vi "Gaussian.vi"() -> ()   [LabVIEW 2011]
uses:
  <vilib>/Math Plots/2D Math Plots/2D Error Bar/2D Error Bar XCtrl/2D Error Bar.xctl
  <vilib>/Math Plots/2D Math Plots/2D Error Bar/2D Error Bar Datatype/Public/Plot Helper (Fixed).vi
  <vilib>/Math Plots/2D Math Plots/2D Error Bar/2D Error Bar Datatype/Public/Plot Helper (Percentage).vi
  <vilib>/Analysis/NI_AALPro.lvlib
  <vilib>/Math Plots/2D Math Plots/2D Error Bar/2D Error Bar Datatype/2D Error Bar Datatype.lvclass
panel:
  in  "y-error (or above)":dbl[](array[numeric])
  in  "x-error (or below)":dbl[](array[numeric])
  out "2D Error Bar":refnum<class "2D Plot Datatype.lvclass">[](xcontrol)
  in  "Array - Numeric":dbl[][](array[numeric])
  out "XY Graph":T1(graph)
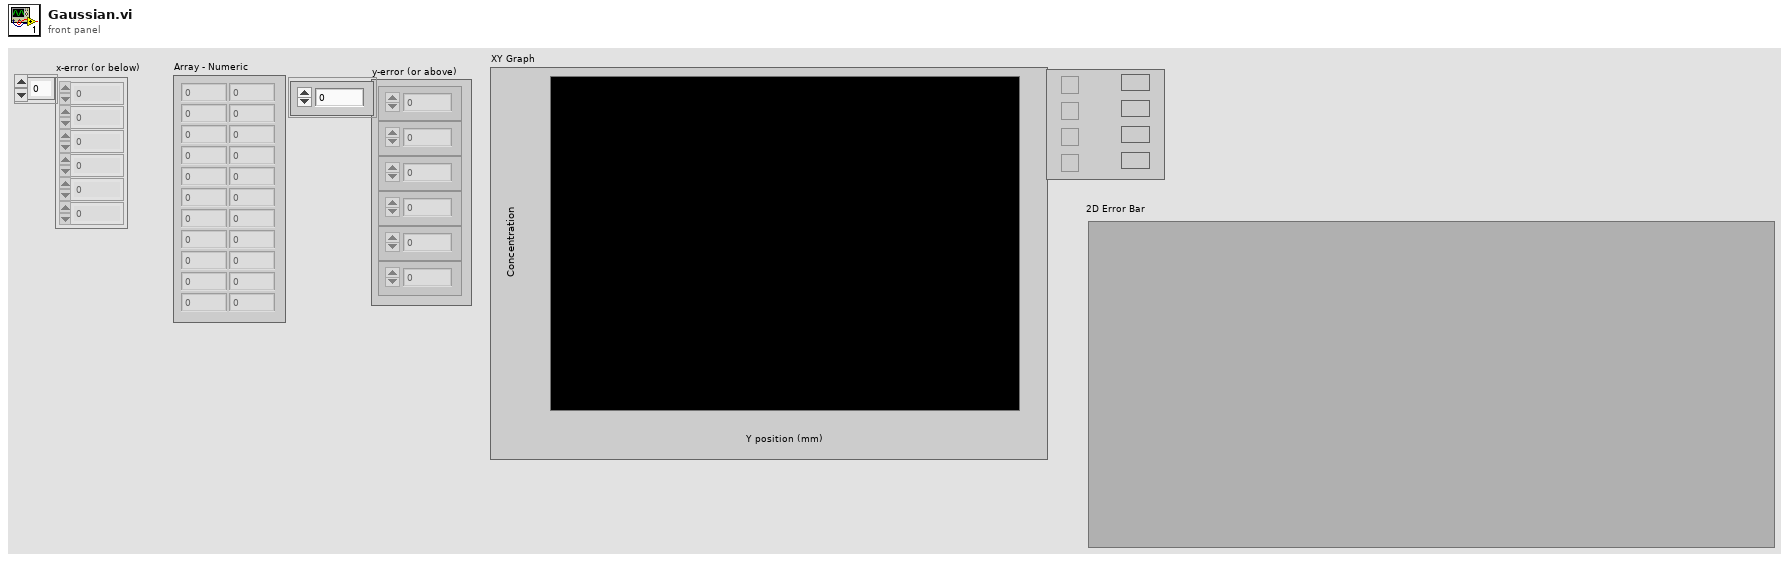
[diagram p1: front panel]
types:
  T1 = cluster{"Array - Numeric":dbl[], "Array - Numeric":dbl[]}[]
  T2 = cluster{"Array - Numeric":dbl[], "Array - Numeric":dbl[]}
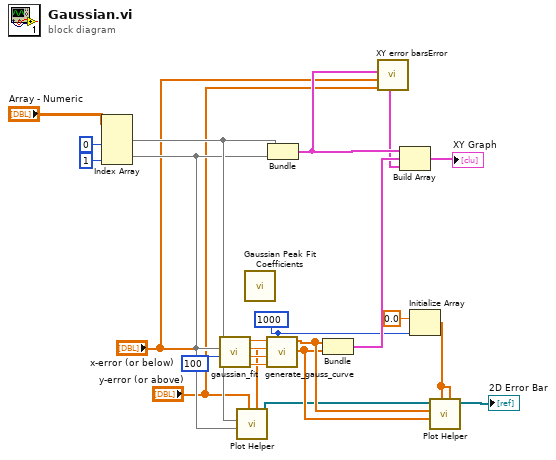
[diagram p0: block diagram]
diagram:
  w7 = 1000
  n1 = Index Array(array="Array - Numeric", index (col) #1=0 ("disabled index (col)"), index (col) #2=1 ("index (col)")) -> (element #1=w9:dbl[], element #2=w8:dbl[])  [unwired: 2 in]
  n2 = call "gaussian_fit.vi"("Max Itterations"=100, "Y Values"=w8, "X Values"=w9) -> ("offset"=w15:dbl, "Spread (st dev)"=w16:dbl, "Center"=w17:dbl, "Amplitude"=w18:dbl)  [unwired: 1 in, 2 out]
  n3 = call-poly <vilib>:"Plot Helper.vi"("error b vector"="x-error (or below)", "error a vector"="y-error (or above)", "y vector"=w8, "x vector"=w9) -> ("2D Plot Class Obj Array out"=w10:refnum<class "2D Plot Datatype.lvclass">[])  [unwired: 2 in, 5 out]
  n4 = call <vilib>:"Gaussian Peak Fit Coefficients.vi"() -> ()  [unwired: 12 in, 4 out]
  n5 = call "generate_gauss_curve.vi"("num points"=w7, "offset"=w15, "Spread"=w16, "Center"=w17, "Amplitude"=w18) -> ("Y Values"=w11:dbl[], "X Values"=w12:dbl[])  [unwired: 3 in]
  n6 = Bundle("Array - Numeric"=w9, "Array - Numeric"=w8) -> (w4:T2)  [unwired: 1 in]
  n7 = Bundle("X Values"=w12, "Y Values"=w11) -> (w14:cluster{"X Values":dbl[], "Y Values":dbl[]})  [unwired: 1 in]
  n8 = call "XY error barsError.vi"("XY plot"=w4, "Xerror"="x-error (or below)", "Yerror"="y-error (or above)") -> ("X+Y error bars"=w3:cluster{dbl[], dbl[]})  [unwired: 5 in, 2 out]
  n9 = Build Array(w4, w14, w3) -> (→"XY Graph":cluster{"X Values":dbl[], "Y Values":dbl[]}[])
  n10 = Initialize Array(0.0 ("element"), w7) -> (w5:dbl[])
  n11 = call-poly <vilib>:"Plot Helper.vi"("error b percentage"=w5, "error a percentage"=w5, "y vector"=w11, "x vector"=w12, "2D Plot Class Obj Array in"=w10) -> ("2D Plot Class Obj Array out"=→"2D Error Bar":refnum<class "2D Plot Datatype.lvclass">[])  [unwired: 1 in, 5 out]
